vi "DigDelay  Test.vi"() -> ()   [LabVIEW 2017]
panel:
  in  "Init":bool
  out "output array":bool[](array[boolean])
  out "subarray":bool[](array[boolean])
  in  "in":bool[](array[boolean])
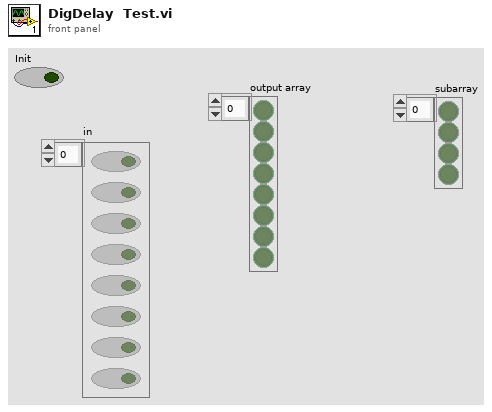
[diagram p1: front panel]
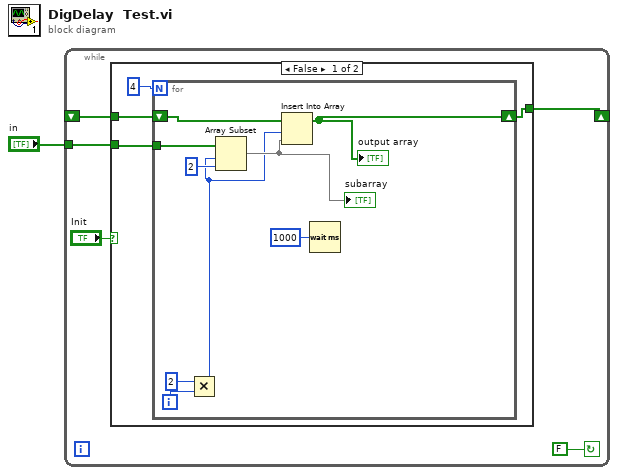
[diagram p0: block diagram]
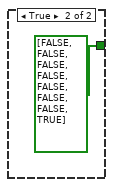
[diagram p2: hidden frame]
diagram:
  n1 = while {
    tunnel: "in" -> [w6]
    shift-right: [w3] -> _
    shift-left: _ -> [w4]
    stop <- FALSE continue-if-true
    n2 = case shown="False" "Init" {
      tunnel: w6 -> [w9 _]
      tunnel: w4 -> [w8 _]
      tunnel: [w7 bool[] [FALSE, FALSE, FALSE, FALSE, FALSE, FALSE, FALSE, TRUE]] -> w3
      frame False {
        n3 = for {
          N: 4 -> [_]
          tunnel: w9 -> [w12]
          shift-right: [w11] -> w7
          shift-left: w8 -> [w13]
          i -> [w19]
          n4 = Multiply(x=2, y=w19) -> (x*y=w15:i32)
          n5 = Array Subset(array=w12, index=w15, length=2) -> (w16:bool[])
          "subarray" <- w16
          n6 = Insert Into Array(array=w13, index=w15, new element=w16) -> (w11:bool[])
          "output array" <- w11
          n7 = Wait (ms)(milliseconds to wait=u32 1000) -> ()  [unwired: 1 out]
        }
      }
      frame True {
      }
    }
  }
